vi "Voltage inquiry.vi"(7 "Channel  (1: CH1)":u16(ring)=1 items=["CH1"=1, "CH2"=2, "CH3"=3, "CH4"=4], 8 "error in (no error)":errorcluster, 11 "VISA resource name":refnum<visa-resource-name>) -> (0 "error out":errorcluster, 2 "Voltage":dbl, 3 "VISA resource name out":refnum<visa-resource-name>)   [LabVIEW 2020, in "GPP.lvlib"]
uses:
  GPP.lvlib
  Function/VISA_COMMON.ctl
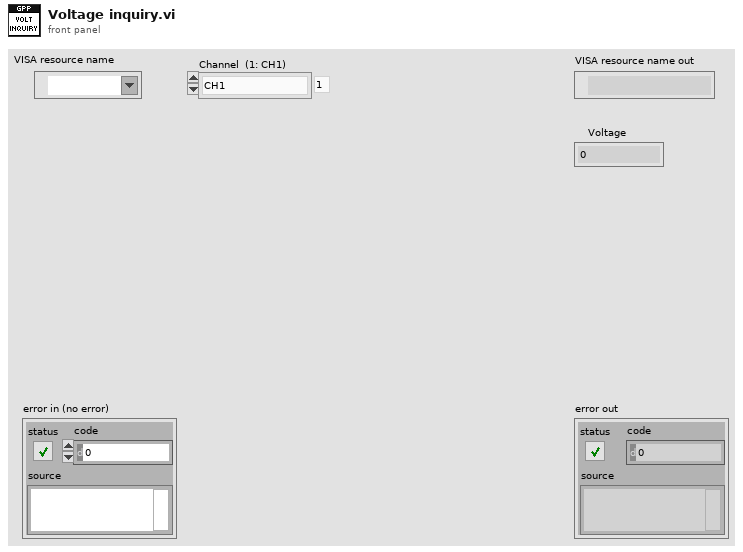
[diagram p1: front panel]
types:
  T1 = typedef "GPP.lvlib/VISA_COMMON.ctl" = enum16{"Initial", "Write CMD", "Read Result", "Read History", "Close"}
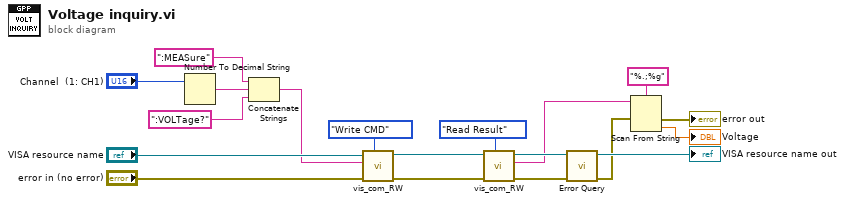
[diagram p0: block diagram]
diagram:
  n1 = Number To Decimal String(number="Channel  (1: CH1)") -> (decimal integer string=w19:string)  [unwired: 1 in]
  n2 = Concatenate Strings(":MEASure", w19, ":VOLTage?") -> (w2:string)
  n3 = call "vis_com_RW.vi"("Funciton"=VISA_COMMON."Write CMD", "error in (no error)"="error in (no error)", "CMD String"=w2, "VISA resource in"="VISA resource name") -> ("error out"=w11:errorcluster, "VISA resource out"=w10:refnum<visa-resource-name>)  [unwired: 5 in, 1 out]
  n4 = call "vis_com_RW.vi"("Funciton"=VISA_COMMON."Read Result", "error in (no error)"=w11, "VISA resource in"=w10) -> ("error out"=w7:errorcluster, "Result"=w8:string, "VISA resource out"=w9:refnum<visa-resource-name>)  [unwired: 6 in]
  n5 = call "Error Query.vi"("error in (no error)"=w7, "VISA resource name"=w9) -> ("error out"=w6:errorcluster, "VISA resource name out"=→"VISA resource name out":refnum<visa-resource-name>)  [unwired: 6 in, 2 out]
  n6 = Scan From String(format string="%.;%g", input string=w8, error in=w6) -> (error out=→"error out":errorcluster, output 1=→"Voltage":dbl)  [unwired: 2 in, 2 out]
